vi "Memory.Pointer.Parameter Check.Length.vi"(7 "calling vi name":string, 8 "error in (no error)":errorcluster, 10 "length":u64 format="%d bytes", 11 "Pointer in":refnum<class "Memory.Pointer.Void.lvclass">) -> (0 "error out":errorcluster, 2 "length out":u64 format="%d bytes", 3 "Pointer out":refnum<class "Memory.Pointer.Void.lvclass">)   [LabVIEW 2016, in "Memory Manager.lvlib" / "Memory.Pointer.Void.lvclass"]
uses:
  Memory.Pointer.Void.lvclass
  Pointer/Memory.Pointer.lvclass
  Typedefs/Memory.Pointer.Parameters.ctl
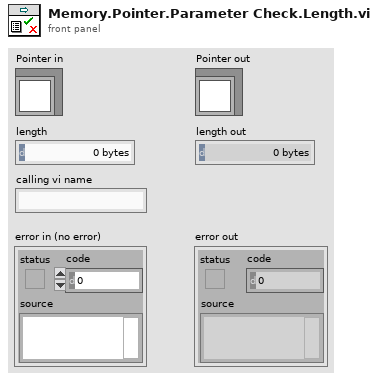
[diagram p1: front panel]
types:
  T1 = typedef "Memory Manager.lvlib/Memory.Pointer.Void.lvclass/Memory.Pointer.Parameters.ctl" = enum16{"offset", "length", "size", "subset"}
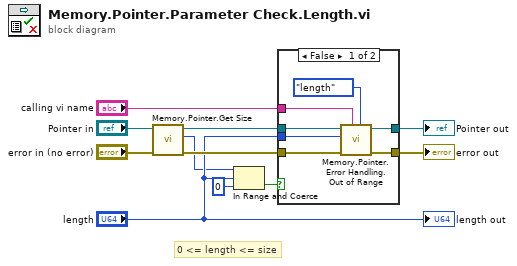
[diagram p0: block diagram]
diagram:
  # "0 <= length <= size"
  n1 = call "Memory.Pointer.Get Size.vi"("error in (no error)"="error in (no error)", "Pointer in"="Pointer in") -> ("error out"=w4:errorcluster, "size"=w1:u64, "Pointer out"=w11:refnum<class "Memory.Pointer.Void.lvclass">)  [unwired: 7 in]
  n2 = In Range and Coerce(upper limit=w1, x="length", lower limit=u64 0) -> (In Range?=w8:bool)  [unwired: 1 out]
  n3 = case shown="False" w8 {
    tunnel: [w18 w20] -> w7
    tunnel: "calling vi name" -> [w17 _]
    tunnel: w4 -> [w16 w20]
    tunnel: "length" -> [w14 _]
    tunnel: w11 -> [w13 w19]
    tunnel: [w12 w19] -> w2
    frame False {
      n4 = call "Memory.Pointer.Error Handling.Out of Range.vi"("parameter"=Memory.Pointer.Parameters."length", "source vi name"=w17, "error in (no error)"=w16, "value"=w14, "Pointer in"=w13) -> ("error out"=w18:errorcluster, "Pointer out"=w12:refnum<class "Memory.Pointer.Void.lvclass">)  [unwired: 5 in]
    }
    frame True {
    }
  }
  "error out" <- w7
  "Pointer out" <- w2
  "length out" <- "length"
